vi "Swift.ProcCases.vi"(0 "i ref in":refnum<vi>, 1 "selector":string, 2 "Data":T1, 3 "call cluster":T2={"Object"="", "Selector"="", "CallType"=enum."synchronous", "Async Object"="", "Async Selector"="", "Data Descriptor"="", "Data"=[], "Error #"=0, "Expire"=0}, 5 "error in (no error)":errorcluster) -> (14 "i ref out":refnum<vi>, 17 "answer cluster":T2={"Object"="", "Selector"="", "CallType"=enum."synchronous", "Async Object"="", "Async Selector"="", "Data Descriptor"="", "Data"=[], "Error #"=0, "Expire"=0}, 19 "error out":errorcluster)   [LabVIEW 2014, in "Swift.lvlib"]
doc: "This method is called by a process from within the default case in the event loop. The methods of a class that are linked to events will be called from THIS method. Add your code here."
uses:
  Swift.lvlib
  CSCore/CSSystem/CoreDefs/CoreDefs.call_type.ctl
  CSCore/BaseProcess/BaseProcess.descriptor string definition.ctl
  CSCore/CSSystem/CoreDefs/CoreDefs.rawDataType.ctl
  CSCore/BaseProcess/BaseProcess.lvlib
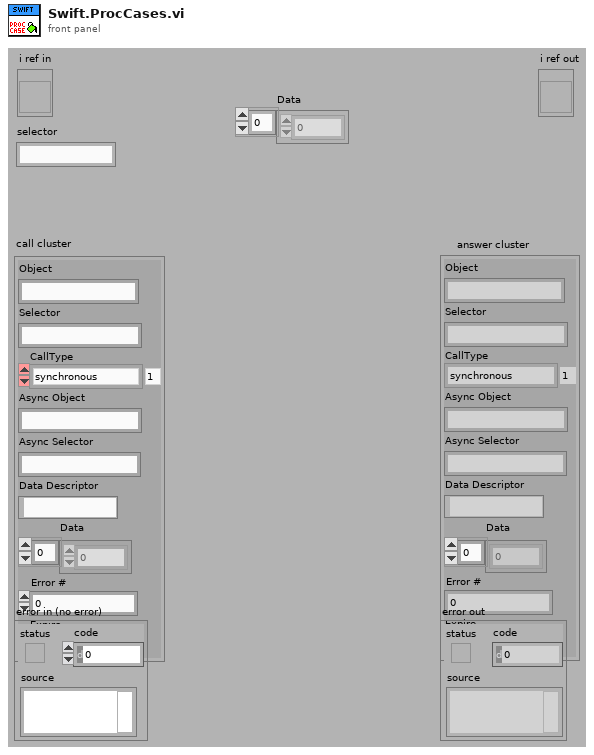
[diagram p1: front panel]
types:
  T1 = typedef "CoreDefs.rawDataType.ctl" = i8[]
  T2 = typedef "CoreDefs.call_type.ctl" = cluster{"Object":string, "Selector":string, "CallType":enum16{"simple", "synchronous", "asynchronous"}, "Async Object":string, "Async Selector":string, "Data Descriptor":T3, "Data":T1, "Error #":i32, "Expire":u32}
  T3 = typedef "BaseProcess.lvlib/BaseProcess.descriptor string definition.ctl" = string
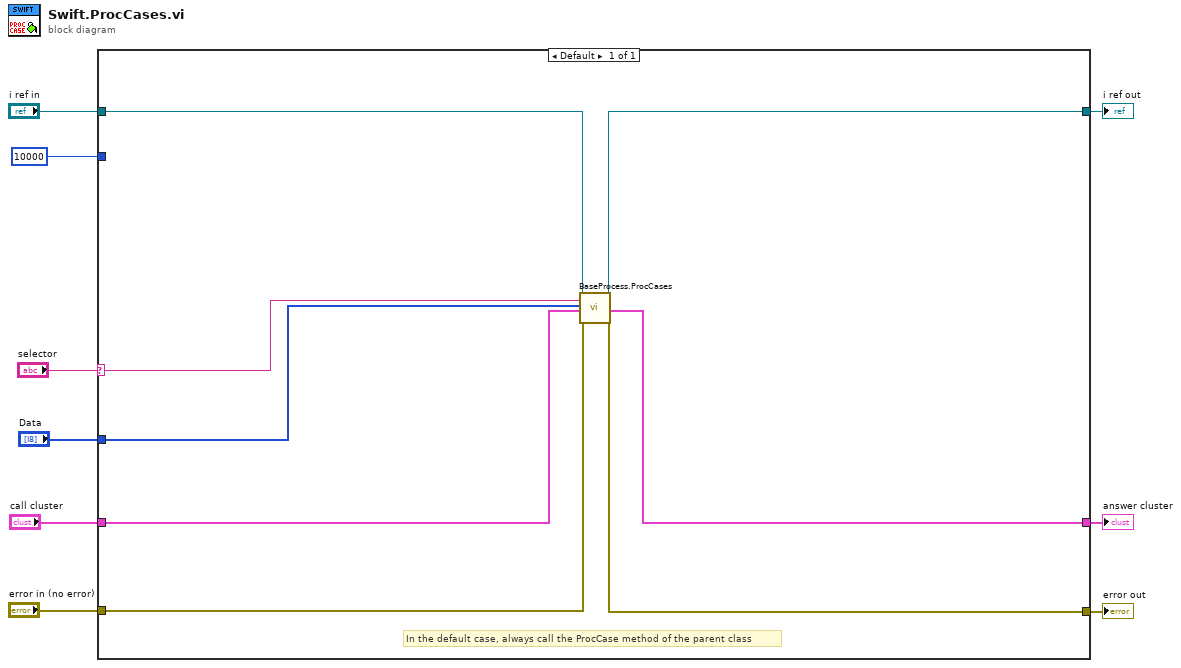
[diagram p0: block diagram]
diagram:
  n1 = case shown="Default" "selector" {
    selector: "selector" -> [w12]
    tunnel: "i ref in" -> [w11]
    tunnel: [w17] -> w5
    tunnel: "call cluster" -> [w13]
    tunnel: [w14] -> w8
    tunnel: "error in (no error)" -> [w16]
    tunnel: [w15] -> w3
    tunnel: 10000 ("ms timeout (100)") -> [_]
    tunnel: "Data" -> [w10]
    frame Default {
      # "In the default case, always call the ProcCase method of the parent class"
      n2 = call "BaseProcess.ProcCases.vi"("i ref in"=w11, "selector"=w12, "Data"=w10, "call cluster"=w13, "error in (no error)"=w16) -> ("i ref out"=w17:refnum<vi>, "answer cluster"=w14:T2, "error out"=w15:errorcluster)  [unwired: 12 in]
    }
  }
  "answer cluster" <- w8
  "i ref out" <- w5
  "error out" <- w3
